vi "GetLasrError.vi"(8 "error in (no error)":errorcluster, 11 "GRMActor in":refnum<class "GRMActor.lvclass">) -> (0 "error out":errorcluster, 2 "LasrError":string, 3 "GRMActor out":refnum<class "GRMActor.lvclass">)   [LabVIEW 2020, in "GRMActor.lvlib" / "GRMActor.lvclass"]
uses:
  GRMActor.lvclass
  GRMActor.lvclass/GRMActor.ctl
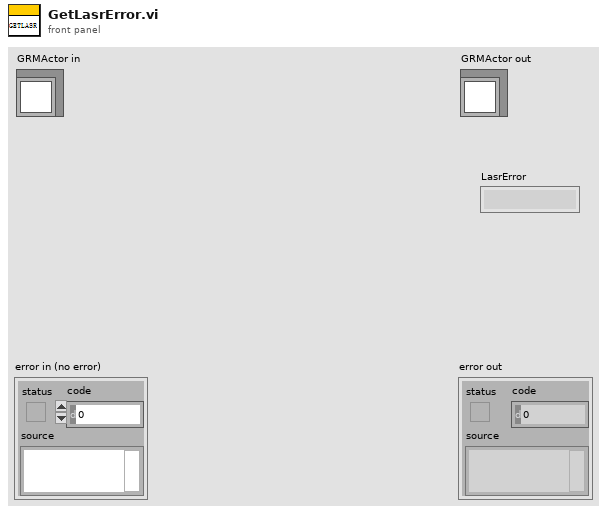
[diagram p1: front panel]
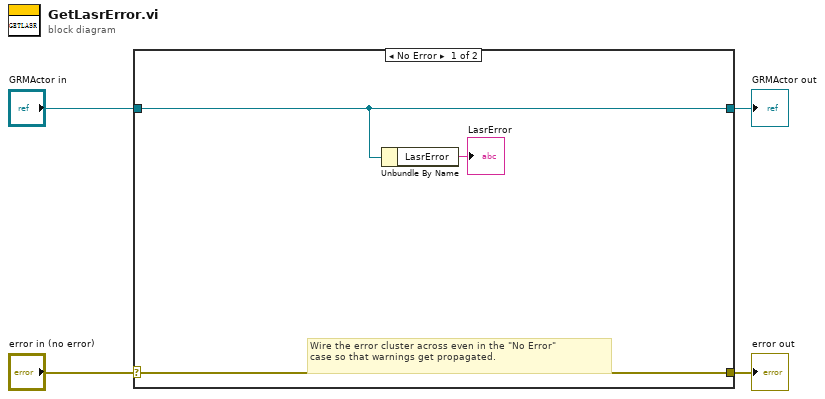
[diagram p0: block diagram]
diagram:
  n1 = case shown="No Error" "error in (no error)" {
    selector: "error in (no error)" -> [w7 w9]
    tunnel: [w7 w9] -> w3
    tunnel: [w6 w8] -> w1
    tunnel: "GRMActor in" -> [w6 w8]
    frame No Error {
      # "Wire the error cluster across even in the \"No Error\"\ncase so that warnings get propagated."
      n2 = Unbundle By Name(w6) -> ("LasrError"=→"LasrError":string)
    }
    frame Error {
    }
  }
  "error out" <- w3
  "GRMActor out" <- w1
